vi "Shooter.vi"(8 "Boolean 2":bool, 9 "Boolean":bool, 10 "Power":dbl, 11 "Motor Ref":string="My Motor RefNum") -> ()   [LabVIEW 2014]
panel:
  in  "Numeric":dbl
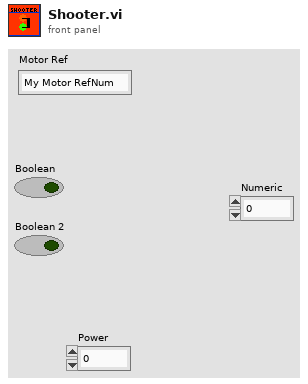
[diagram p1: front panel]
types:
  T1 = typedef "WPI_MotorControlDeviceRef.ctl" = cluster{"DeviceStatus":errorcluster, "Type":T2, "PWM":cluster{"Controller":T3, "PWM Channel":T4, "DeadBand":T5}, "CAN":cluster{"Device Number":u8, "Control Mode":T6, "Semaphore":T7, "Max Vout":dbl, "TalonSRX Control Mode":T8}, "Invert":bool, "TransformRef":T9, "InvTransformRef":T9}
  T2 = typedef "WPI_MotorControlType.ctl" = enum16{"PWM", "CAN", "CANTalonSRX"}
  T3 = typedef "FPGA_TypedefDigitalModule.ctl" = enum16{"Controller 1"}
  T4 = typedef "FPGA_DIOPWMChannel.ctl" = enum8{"PWM 0", "PWM 1", "PWM 2", "PWM 3", "PWM 4", "PWM 5", "PWM 6", "PWM 7", "PWM 8", "PWM 9", "PWM MXP 0", "PWM MXP 1", "PWM MXP 2", "PWM MXP 3", "PWM MXP 4", "PWM MXP 5", "PWM MXP 6", "PWM MXP 7", "PWM MXP 8", "PWM MXP 9", "Invalid"}
  T5 = typedef "WPI_PWMDeadband.ctl" = cluster{"Name":string, "maxPositivePwm":i32, "minPositivePwm":i32, "centerPwm":i32, "maxNegativePwm":i32, "minNegativePwm":i32, "angularRange":u16}
  T6 = typedef "WPI_CANJaguar_ControlMode.ctl" = enum8{"Percent VBus", "Current", "Speed", "Position", "Voltage"}
  T7 = typedef "Semaphore RefNum" = refnum<k1>
  T8 = typedef "WPI_CANTalonSRX_APIControlMode.ctl" = enum8{"Percent VBus", "Speed", "Position", "Slave", "Unchanged / Invalid"}
  T9 = typedef "WPI_PWMTransform_ConPane.ctl" = refnum<vi>
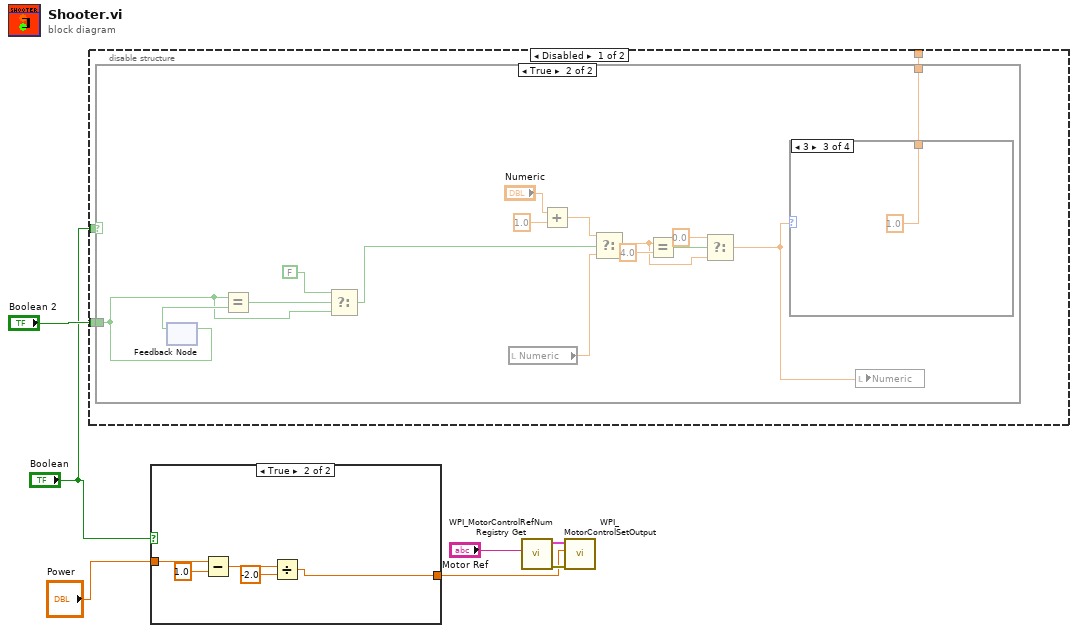
[diagram p0: block diagram]
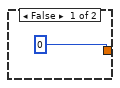
[diagram p2: hidden frame]
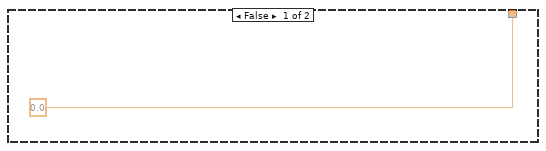
[diagram p3: hidden frame]
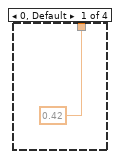
[diagram p4: hidden frame]
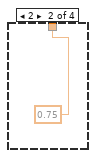
[diagram p5: hidden frame]
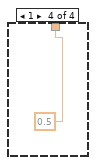
[diagram p6: hidden frame]
diagram:
  n1 = disable-structure shown="Disabled" {
    disable-tunnel: "Boolean 2" -> [w10 _]
    disable-tunnel: "Boolean" -> [w9 _]
    disable-tunnel: [w8 _] -> _
    frame Disabled {
      n2 = case shown="True" w9 {
        tunnel: w10 -> [_ w12]
        tunnel: [0.0 ("Output") w17] -> w8
        frame False {
        }
        frame True {
          n3 = feedback-in #1(w12) -> ()
          n4 = feedback #1() -> (w16:bool)  [unwired: 1 in]
          n5 = Equal?(x=w12, y=w16) -> (x = y?=w15:bool)
          n6 = Select(t=FALSE ("Boolean 2"), s=w15, f=w12) -> (s? t:f=w14:bool)
          n7 = local read "Numeric"() -> (w23:dbl)
          n8 = Add(x="Numeric", y=1.0) -> (x+y=w26:dbl)
          n9 = Select(t=w26, s=w14, f=w23) -> (s? t:f=w18:dbl)
          n10 = Equal?(x=w18, y=4.0) -> (x = y?=w21:bool)
          n11 = Select(t=0.0, s=w21, f=w18) -> (s? t:f=w20:dbl)
          n12 = case shown="3" w20 {
            tunnel: [0.42 ("Output") 0.75 ("Output") 1.0 ("Output") 0.5 ("Output")] -> w17
            frame 0, Default {
            }
            frame 2 {
            }
            frame 3 {
            }
            frame 1 {
            }
          }
          n13 = local write "Numeric"(w20) -> ()
        }
      }
    }
    frame Enabled {
    }
  }
  n14 = case shown="True" "Boolean" {
    tunnel: "Power" -> [_ w36]
    tunnel: [0 w32] -> w1
    frame False {
    }
    frame True {
      n15 = Subtract(x=w36, y=1.0) -> (x-y=w34:dbl)
      n16 = Divide(x=w34, y=-2.0) -> (x/y=w32:dbl)
    }
  }
  n17 = call <vilib>:"WPI_MotorControlRefNum Registry Get.vi"("refnum name"="Motor Ref") -> ("error out"=w7:errorcluster, "MotorControlDevRef"=w6:T1)  [unwired: 9 in]
  n18 = call <vilib>:"WPI_MotorControlSetOutput.vi"("error in (no error)"=w7, "Output"=w1, "MotorControlDevRef"=w6) -> ()  [unwired: 6 in, 3 out]
